vi "Cancel Event Wait.vi"(3 "error in (no error)":errorcluster, 4 "ExecAnchor in":refnum<class "ExecAnchor.lvclass">) -> (0 "error out":errorcluster)   [LabVIEW 2020, in "ExecAnchor.lvclass"]
uses:
  ExecAnchor.lvclass
  ExecAnchor.lvclass/ExecAnchor.ctl
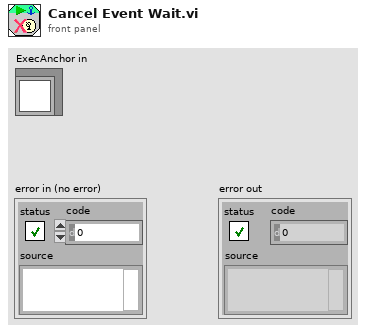
[diagram p1: front panel]
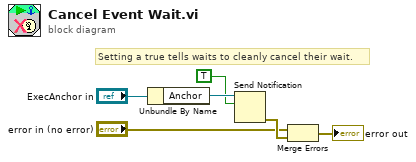
[diagram p0: block diagram]
diagram:
  # "Setting a true tells waits to cleanly cancel their wait."
  n1 = Unbundle By Name("ExecAnchor in") -> ("Anchor"=w5:refnum<notifier>)
  n2 = Send Notification(notification=TRUE ("element"), notifier=w5) -> (error out=w4:errorcluster)  [unwired: 1 in, 1 out]
  n3 = Merge Errors("error in (no error)", w4) -> (→"error out":errorcluster)
